vi "Get Data From Excel.vi"(8 "error in (no error)":errorcluster, 11 "NI Generic Parser in":refnum<class "NI Generic Parser.lvclass">=refnum) -> (0 "error out":errorcluster, 3 "NI Generic Parser out":refnum<class "NI Generic Parser.lvclass">)   [LabVIEW 2018, in "NI Generic Parser.lvlib" / "NI Generic Parser.lvclass"]
uses:
  NI Generic Parser.lvclass
  <vilib>/addons/_office/NI_ReportGenerationToolkit.lvlib
  <vilib>/Utility/NIReport.llb/NI_report.lvclass
  <vilib>/addons/_office/excel.llb/Excel Get Data ([str]).vi
  <vilib>/Utility/NIReport.llb/Excel/NI_Excel.lvclass
  Controls/WorkSheet Data.ctl
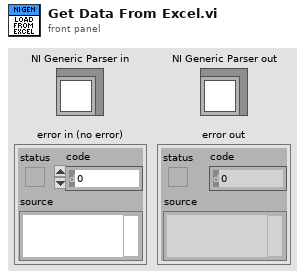
[diagram p1: front panel]
types:
  T1 = enum16{"Standard Report", "HTML", "Word", "Excel"}
  T2 = typedef "NI Generic Parser.lvlib/NI Generic Parser.lvclass/WorkSheet Data.ctl" = cluster{"Worksheet Name":string, "Worksheet Data":string[][]}
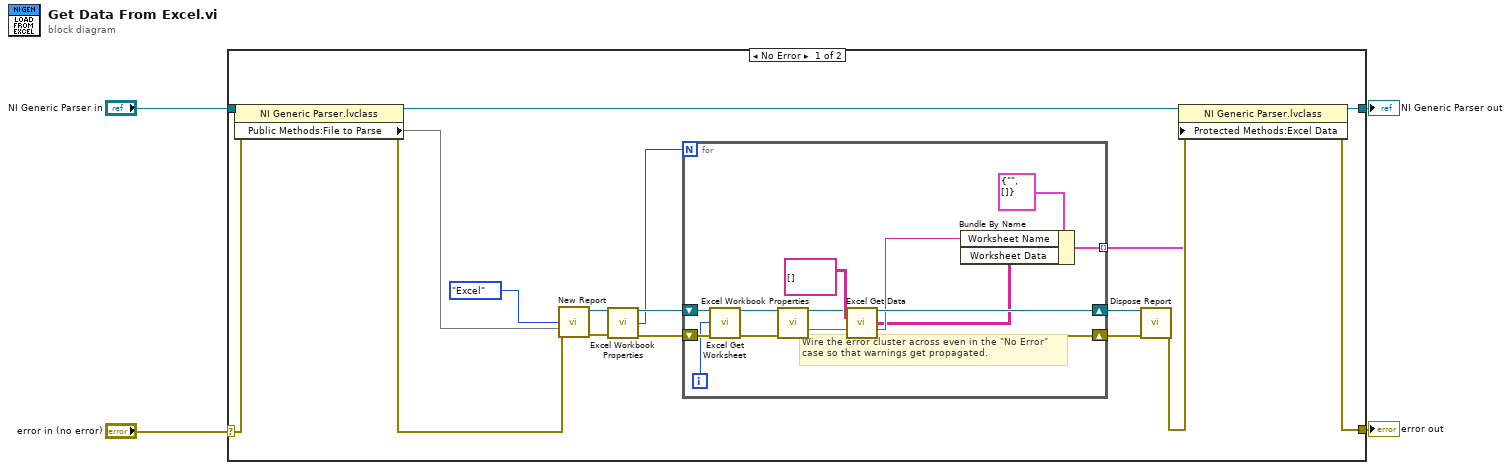
[diagram p0: block diagram]
diagram:
  n1 = case shown="No Error" "error in (no error)" {
    selector: "error in (no error)" -> [w21 w37]
    tunnel: [w6 w37] -> w3
    tunnel: [w8 w36] -> w1
    tunnel: "NI Generic Parser in" -> [w20 w36]
    frame No Error {
      # "Wire the error cluster across even in the \"No Error\"\ncase so that warnings get propagated."
      n2 = property class="NI Generic Parser.lvclass"(reference=w20, error in=w21) -> (reference out=w9:refnum<class "NI Generic Parser.lvclass">, error out=w11:errorcluster, "Public Methods:File to Parse"=w10)
      n3 = call <vilib>:"New Report.vi"("report type"=T1."Excel", "template (empty)"=w10, "error in (no error)"=w11) -> ("report out"=w18:refnum<class "NI_report.lvclass">, "error out"=w17:errorcluster)  [unwired: 11 in]
      n4 = call <vilib>:"Excel Workbook Properties.vi"("report in"=w18, "error in (no error)"=w17) -> ("report out"=w13:refnum<class "NI_report.lvclass">, "worksheets count"=w12:i32, "error out"=w16:errorcluster)  [unwired: 10 in, 1 out]
      n5 = for {
        N: w12 -> [_]
        shift-right: [w33] -> w14
        shift-left: w16 -> [w35]
        shift-right: [w34] -> w15
        shift-left: w13 -> [w31]
        tunnel: [w23] -> w5 mode=indexing
        i -> [w30]
        n6 = call <vilib>:"Excel Get Worksheet.vi"("report in"=w31, "worksheet index (0)"=w30, "error in (no error)"=w35) -> ("report out"=w27:refnum<class "NI_report.lvclass">, "error out"=w32:errorcluster)  [unwired: 11 in]
        n7 = call <vilib>:"Excel Workbook Properties.vi"("report in"=w27, "error in (no error)"=w32) -> ("report out"=w26:refnum<class "NI_report.lvclass">, "current worksheet name"=w25:string, "error out"=w28:errorcluster)  [unwired: 10 in, 1 out]
        n8 = call-poly <vilib>:"Excel Get Data.vi"("report in"=w26, "data type"=string[][] [], "error in (no error)"=w28) -> ("report out"=w34:refnum<class "NI_report.lvclass">, "data"=w24:string[][], "error out"=w33:errorcluster)  [unwired: 10 in]
        n9 = Bundle By Name(cluster=T2 {"Worksheet Name"="", "Worksheet Data"=[]} ("Worksheet Data"), "Worksheet Name"=w25, "Worksheet Data"=w24) -> (w23:T2)
      }
      n10 = call-dynamic "Dispose Report.vi"("report in"=w15, "error in (no error)"=w14) -> ("error out"=w7:errorcluster)  [unwired: 13 in]
      n11 = property class="NI Generic Parser.lvclass"(reference=w9, error in=w7, "Protected Methods:Excel Data"=w5) -> (reference out=w8:refnum<class "NI Generic Parser.lvclass">, error out=w6:errorcluster)
    }
    frame Error {
    }
  }
  "error out" <- w3
  "NI Generic Parser out" <- w1
